vi "test5-AsyncMessageWithReply.vi"(8 "error in (no error)":errorcluster, 11 "TestCase in":refnum<class "testcase-CSMMessage.lvclass">) -> (0 "error out":errorcluster, 3 "TestCase out":refnum<class "testcase-CSMMessage.lvclass">)   [LabVIEW 2017, in "testcase-CSMMessage.lvclass"]
uses:
  testcase-CSMMessage.lvclass
  7412589e-de49-4983-aece-358686b48526.vi
  src/user.lib/_NEVSTOP/Communicable State Machine(CSM)/AdvanceAPI/CSM - Make String Arguments Safe.vi
  src/user.lib/_NEVSTOP/Communicable State Machine(CSM)/AdvanceAPI/CSM - Keywords.vi
  <vilib>/addons/_JKI Toolkits/VI Tester/TestCase.llb/TestCase.lvclass
  src/user.lib/_NEVSTOP/Communicable State Machine(CSM)/Communicable State Machine.lvlib
  C:/Program Files (x86)/National Instruments/LabVIEW 2017/vi.lib/addons/_JKI Toolkits/VI Tester/TestCase.llb/TestCase.lvclass
panel:
  out "Loop count":i32
  out "debug message":string
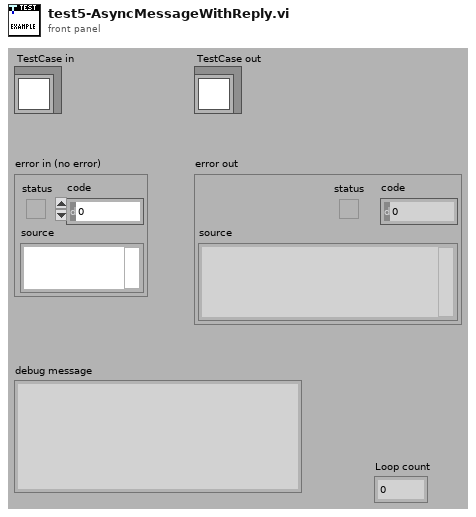
[diagram p1: front panel]
types:
  T1 = cluster{"Arguments":string, "Response":string, "error":errorcluster}
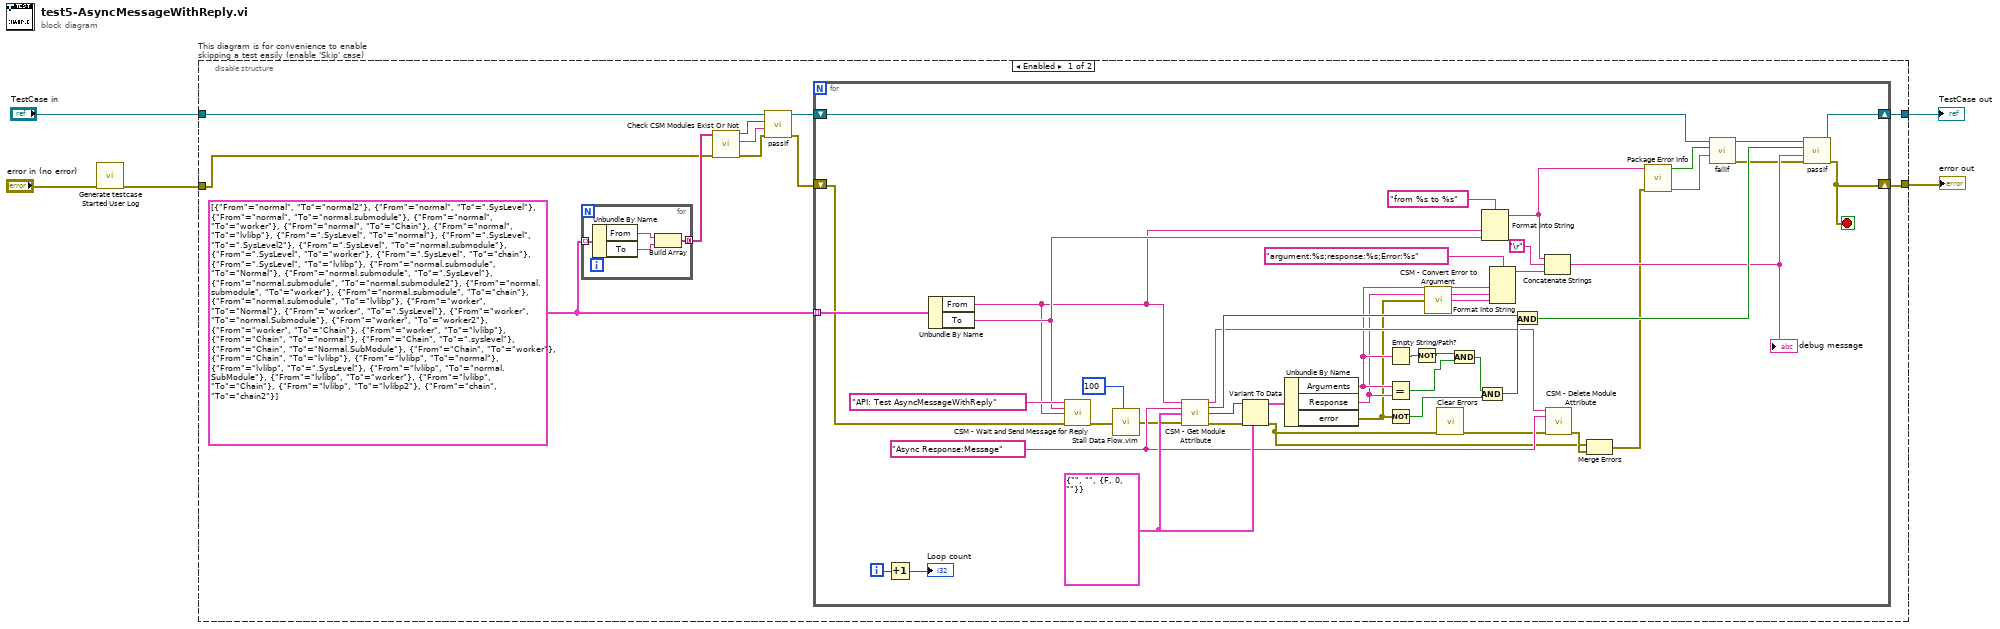
[diagram p0: block diagram]
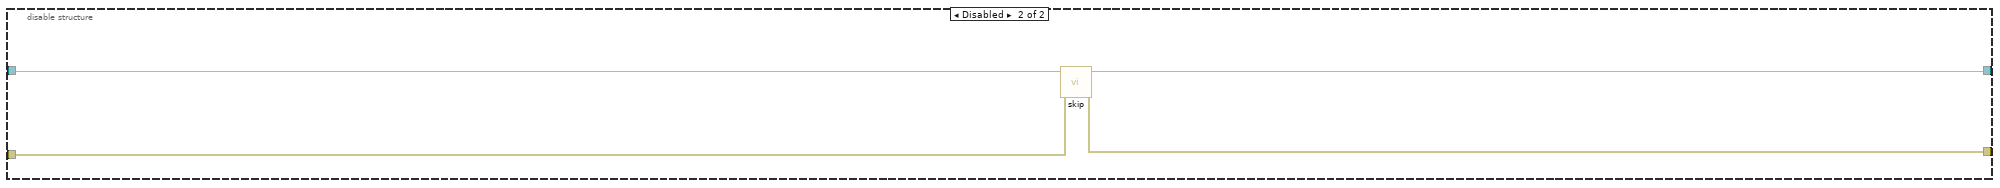
[diagram p2: hidden frame]
diagram:
  n1 = call "Generate testcase Started User Log.vi"("Error In"="error in (no error)") -> ("error out"=w1:errorcluster)  [unwired: 10 in]
  n2 = disable-structure "This diagram is for convenience to enable skipping a test easily (enable 'Skip' case)" shown="Enabled" {
    disable-tunnel: "TestCase in" -> [w9 w69]
    disable-tunnel: [w7 w67] -> w2
    disable-tunnel: [w6 w68] -> w4
    disable-tunnel: w1 -> [w10 w66]
    frame Enabled {
      w12 = cluster{"From":string, "To":string}[] [{"From"="normal", "To"="normal2"}, {"From"="normal", "To"=".SysLevel"}, {"From"="normal", "To"="normal.submodule"}, {"From"="normal", "To"="worker"}, {"From"="normal", "To"="Chain"}, {"From"="normal", "To"="lvlibp"}, {"From"=".SysLevel", "To"="normal"}, {"From"=".SysLevel", "To"=".SysLevel2"}, {"From"=".SysLevel", "To"="normal.submodule"}, {"From"=".SysLevel", "To"="worker"}, {"From"=".SysLevel", "To"="chain"}, {"From"=".SysLevel", "To"="lvlibp"}, {"From"="normal.submodule", "To"="Normal"}, {"From"="normal.submodule", "To"=".SysLevel"}, {"From"="normal.submodule", "To"="normal.submodule2"}, {"From"="normal.submodule", "To"="worker"}, {"From"="normal.submodule", "To"="chain"}, {"From"="normal.submodule", "To"="lvlibp"}, {"From"="worker", "To"="Normal"}, {"From"="worker", "To"=".SysLevel"}, {"From"="worker", "To"="normal.Submodule"}, {"From"="worker", "To"="worker2"}, {"From"="worker", "To"="Chain"}, {"From"="worker", "To"="lvlibp"}, {"From"="Chain", "To"="normal"}, {"From"="Chain", "To"=".syslevel"}, {"From"="Chain", "To"="Normal.SubModule"}, {"From"="Chain", "To"="worker"}, {"From"="Chain", "To"="lvlibp"}, {"From"="lvlibp", "To"="normal"}, {"From"="lvlibp", "To"=".SysLevel"}, {"From"="lvlibp", "To"="normal.SubModule"}, {"From"="lvlibp", "To"="worker"}, {"From"="lvlibp", "To"="Chain"}, {"From"="lvlibp", "To"="lvlibp2"}, {"From"="chain", "To"="chain2"}]
      n3 = for {
        tunnel: w12 -> [w20] mode=indexing
        tunnel: [w17] -> w15 mode=concatenating
        n4 = Unbundle By Name(w20) -> ("From"=w19:string, "To"=w18:string)
        n5 = Build Array(w19, w18) -> (w17:string[])
      }
      n6 = call "Check CSM Modules Exist Or Not.vi"("error in"=w10, "CSM names in"=w15) -> ("error out"=w13:errorcluster, "Debug string"=w14:string, "All Modules Exist?"=w16:bool)  [unwired: 7 in]
      n7 = call-dynamic "passIf.vi"("error in (no error)"=w13, "message (\"\")"=w14, "pass"=w16, "TestCase in"=w9) -> ("error out"=w11:errorcluster, "TestCase out"=w8:refnum<class "testcase-CSMMessage.lvclass">)  [unwired: 6 in]
      n8 = for {
        tunnel: w12 -> [w55] mode=indexing
        shift-right: [w65] -> w7
        shift-left: w8 -> [w25]
        shift-right: [w38] -> w6
        shift-left: w11 -> [w31]
        i -> [w33]
        stop <- w38 stop-if-true
        w62 = T1 {"Arguments"="", "Response"="", "error"={"status"=FALSE, "code"=0, "source"=""}}
        w51 = "Async Response:Message" ("State")
        n9 = Increment(x=w33) -> (x+1=→"Loop count":i32)
        n10 = Unbundle By Name(w55) -> ("From"=w37:string, "To"=w54:string)
        n11 = call "CSM - Wait and Send Message for Reply.vi"("State"="API: Test AsyncMessageWithReply", "Arguments (\"\")"=w54, "Target Module"=w37, "Error In (No Error)"=w31) -> ("error out"=w35:errorcluster)  [unwired: 8 in, 3 out]
        n12 = call "Stall Data Flow.vim"("value in"=w35, "milliseconds to wait"=u32 100) -> ("value out"=w36:errorcluster)  [unwired: 1 out]
        n13 = call "CSM - Get Module Attribute.vi"("CSM Name"=w37, "Attribute"=w51, "Default Value (Empty Variant)"=w62, "Error In"=w36) -> ("CSM Name (Dup)"=w52:string, "Found"=w58:bool, "Value"=w61:variant, "error out"=w63:errorcluster)  [unwired: 7 in, 1 out]
        n14 = Variant To Data(error in=w63, type=w62, Variant=w61) -> (data=w60:T1, error out=w29:errorcluster)
        n15 = Unbundle By Name(w60) -> ("Arguments"=w46:string, "Response"=w45:string, "error"=w43:errorcluster)
        n16 = Empty String/Path?(string/path=w46) -> (empty?=w50:bool)
        n17 = Equal?(x=w46, y=w45) -> (x = y?=w48:bool)
        n18 = Not(x=w43) -> (.not. x?=w59:bool)
        n19 = Not(x=w50) -> (.not. x?=w49:bool)
        n20 = call "CSM - Convert Error to Argument.vi"("Error"=w43) -> ("Argument"=w44:string)  [unwired: 4 in]
        n21 = call <vilib>:"Clear Errors.vi"("error in (no error)"=w29) -> ("error out"=w39:errorcluster)  [unwired: 5 in, 1 out]
        n22 = And(x=w49, y=w48) -> (x .and. y?=w47:bool)
        n23 = And(x=w47, y=w59) -> (x .and. y?=w57:bool)
        n24 = Format Into String(format string="from %s to %s", w37, w54) -> (resulting string=w21:string)  [unwired: 2 in, 1 out]
        n25 = Format Into String(format string="argument:%s;response:%s;Error:%s", w46, w45, w44) -> (resulting string=w42:string)  [unwired: 2 in, 1 out]
        n26 = And(x=w58, y=w57) -> (x .and. y?=w56:bool)
        n27 = Concatenate Strings(w21, "\r", w42) -> (w28:string)
        "debug message" <- w28
        n28 = call "CSM - Delete Module Attribute.vi"("CSM Name"=w52, "Attribute"=w51, "Error In"=w39) -> ("error out"=w30:errorcluster)  [unwired: 9 in, 3 out]
        n29 = Merge Errors(w29, w30) -> (w22:errorcluster)
        n30 = call "Package Error Info.vi"("error in"=w22, "String in"=w21) -> ("packed error info out"=w26:string, "error status"=w27:bool)  [unwired: 8 in]
        n31 = call-dynamic "failIf.vi"("message (\"\")"=w26, "fail"=w27, "TestCase in"=w25) -> ("error out"=w23:errorcluster, "TestCase out"=w24:refnum<class "testcase-CSMMessage.lvclass">)  [unwired: 7 in]
        n32 = call-dynamic "passIf.vi"("error in (no error)"=w23, "message (\"\")"=w28, "pass"=w56, "TestCase in"=w24) -> ("error out"=w38:errorcluster, "TestCase out"=w65:refnum<class "testcase-CSMMessage.lvclass">)  [unwired: 6 in]
      }
    }
    frame Disabled {
      # "skip test result while test is under development"
      n33 = call <vilib>:"skip.vi"("error in (no error)"=w66, "TestCase in"=w69) -> ("error out"=w68:errorcluster, "TestCase out"=w67:refnum<class "testcase-CSMMessage.lvclass">)  [unwired: 8 in]
    }
  }
  "error out" <- w4
  "TestCase out" <- w2
